vi "GetDriverName.vi"(8 "Error In":errorcluster, 11 "reference in":refnum<class "VdInstrument.lvclass">) -> (0 "Error Out":errorcluster, 2 "DriverName":string, 3 "reference out":refnum<class "VdInstrument.lvclass">)   [LabVIEW 2020, in "VdInstrument.lvclass"]
uses:
  VdInstrument.lvclass
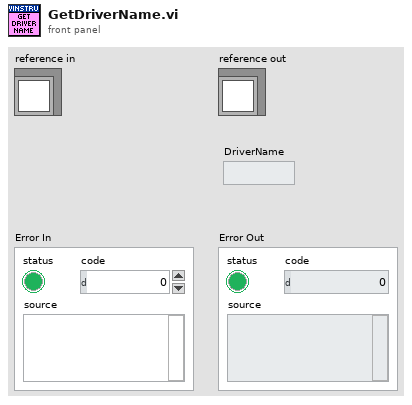
[diagram p1: front panel]
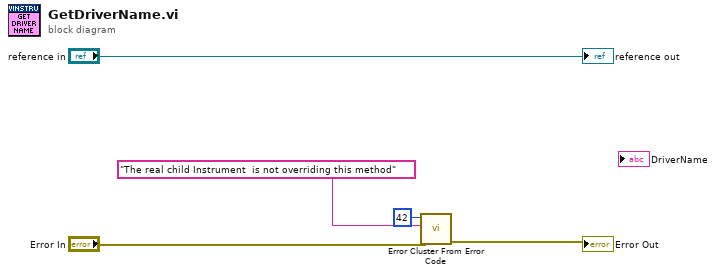
[diagram p0: block diagram]
diagram:
  n1 = call <vilib>:"Error Cluster From Error Code.vi"("error in (no error)"="Error In", "error message (\"\")"="The real child Instrument  is not overriding this method" ("error message (\"\")"), "error code (0)"=42) -> ("error out"=→"Error Out":errorcluster)  [unwired: 6 in]
  "reference out" <- "reference in"
